vi "GV memory address.vi"() -> ()   [LabVIEW 2017]
panel:
  out "Memory addres":cluster{"Boolean":bool, "Numeric":u16}
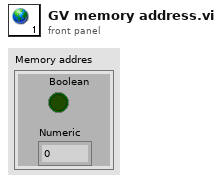
[diagram p1: front panel]
diagram:
